vi "SPIKE <-> PyBd.vi"() -> ()   [LabVIEW 2016]
uses:
  VIs/uPythonX/uPythonX.xctl
panel:
  in  "Spike 2":T1(xcontrol)={"VISA Refnum in"="ASRL73::INSTR", "Python Code"="import hub,utime\n\nhub.port.B.info()\n\n# if info comes back with None - then you have to restart the pybaord\n\nwhile True:\n     try:\n          value = hub.port.B.device.get()[0]\n          # print(value)\n          hub.display.show(str(value))\n          utime.sleep(0.2)\n     except:\n          utime.sleep(1)\n"}
  in  "Spike":T1(xcontrol)={"VISA Refnum in"="ASRL73::INSTR", "Python Code"="import LPF2Class, utime, gc\n\nfrom pyb import LED\n\nred_led   = LED(1)\ngreen_led = LED(2)\nblue_led  = LED(3)\n\n# loop from -10 to 10\ni=0\nred_led.on()\nlpf2 = LPF2Class.LPF2(1, 'Y1', 'Y2')    # PyBD\nlpf2.initialize()\n\nwhile True:\n     if not lpf2.connected:\n          red_led.on()\n          utime.sleep(1)\n          lpf2.initialize()\n     else:\n          red_led.off()\n          while lpf2.connected:\n               gc.collect()\n               lpf2.send_value(i)\n               i += 1\n               # print(lpf2.connected)\n               if i > 10: i=-10\n               utime.sleep_ms(200)\n"}
  # "Do \"Comaprison\" - on both Update and File Save"
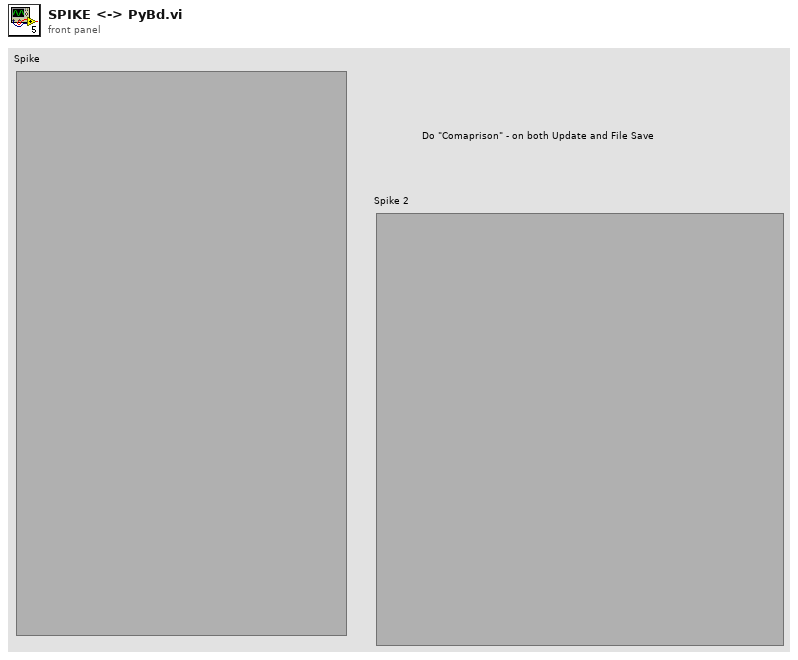
[diagram p1: front panel]
types:
  T1 = cluster{"VISA Refnum in":refnum<visa-resource-name>, "Python Code":string}
  T2 = cluster{"Name":string, "Format":cluster{"# Datasets":u8, "Data Type":u8, "Figures":u8, "Decimals":u8}, "Raw":cluster{"Min":dbl, "Max":dbl}, "Pct":cluster{"Min":dbl, "Max":dbl}, "SI":cluster{"Min":dbl, "Max":dbl}, "Symbol":string, "Funct Map":cluster{"In":u8, "Out":u8}, "view?":bool}[]
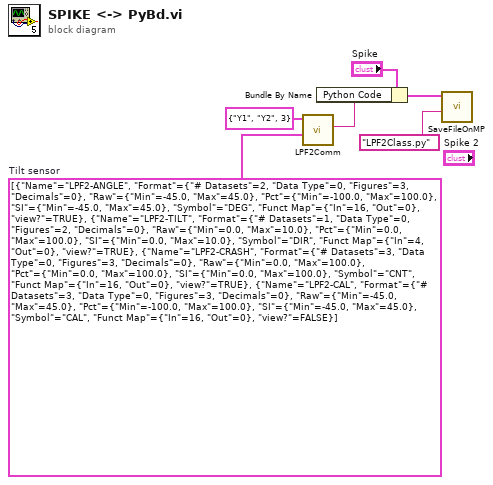
[diagram p0: block diagram]
diagram:
  w5 = T2 [{"Name"="LPF2-ANGLE", "Format"={"# Datasets"=2, "Data Type"=0, "Figures"=3, "Decimals"=0}, "Raw"={"Min"=-45.0, "Max"=45.0}, "Pct"={"Min"=-100.0, "Max"=100.0}, "SI"={"Min"=-45.0, "Max"=45.0}, "Symbol"="DEG", "Funct Map"={"In"=16, "Out"=0}, "view?"=TRUE}, {"Name"="LPF2-TILT", "Format"={"# Datasets"=1, "Data Type"=0, "Figures"=2, "Decimals"=0}, "Raw"={"Min"=0.0, "Max"=10.0}, "Pct"={"Min"=0.0, "Max"=100.0}, "SI"={"Min"=0.0, "Max"=10.0}, "Symbol"="DIR", "Funct Map"={"In"=4, "Out"=0}, "view?"=TRUE}, {"Name"="LPF2-CRASH", "Format"={"# Datasets"=3, "Data Type"=0, "Figures"=3, "Decimals"=0}, "Raw"={"Min"=0.0, "Max"=100.0}, "Pct"={"Min"=0.0, "Max"=100.0}, "SI"={"Min"=0.0, "Max"=100.0}, "Symbol"="CNT", "Funct Map"={"In"=16, "Out"=0}, "view?"=TRUE}, {"Name"="LPF2-CAL", "Format"={"# Datasets"=3, "Data Type"=0, "Figures"=3, "Decimals"=0}, "Raw"={"Min"=-45.0, "Max"=45.0}, "Pct"={"Min"=-100.0, "Max"=100.0}, "SI"={"Min"=-45.0, "Max"=45.0}, "Symbol"="CAL", "Funct Map"={"In"=16, "Out"=0}, "view?"=FALSE}]  # Tilt sensor
  n1 = call "LPF2Comm.vi"("Sensor"=w5, "Pins"=cluster{"Tx":string, "Rx":string, "UART":i8} {"Tx"="Y1", "Rx"="Y2", "UART"=3}) -> ("Python Code"=w3:string)  [unwired: 9 in]
  n2 = Bundle By Name(cluster="Spike", "Python Code"=w3) -> (w2:T1)
  n3 = call "SaveFileOnMP.vi"("FileName"="LPF2Class.py", "VISA in"=w2) -> ()  [unwired: 7 in, 3 out]
